vi "OpenLogs.vi"(8 "error in (no error)":errorcluster, 11 "object in":refnum<class "EventLogger_Actor.lvclass">) -> (0 "error out":errorcluster, 3 "object out":refnum<class "EventLogger_Actor.lvclass">)   [LabVIEW 2014, in "EventLogger_Actor.lvlib" / "EventLogger_Actor.lvclass"]
uses:
  EventLogger_Actor.lvclass
  EventLogger_Actor.lvclass/EventLogger_Actor.ctl
panel:
  # "Connector Pane"
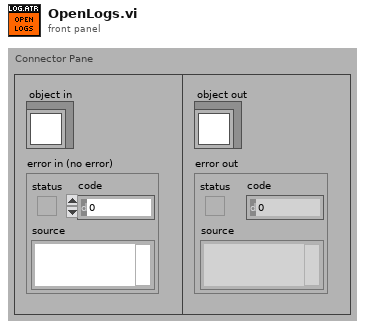
[diagram p1: front panel]
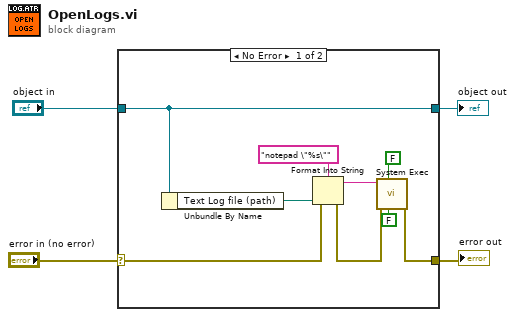
[diagram p0: block diagram]
diagram:
  n1 = case shown="No Error" "error in (no error)" {
    selector: "error in (no error)" -> [w13 w15]
    tunnel: [w11 w15] -> w3
    tunnel: [w12 w14] -> w1
    tunnel: "object in" -> [w12 w14]
    frame No Error {
      n2 = Unbundle By Name(w12) -> ("Text Log file (path)"=w5:path)
      n3 = Format Into String(format string="notepad \"%s\"", error in=w13, w5) -> (resulting string=w8:string, error out=w6:errorcluster)  [unwired: 1 in]
      n4 = call <vilib>:"System Exec.vi"("run minimized? (F)"=FALSE, "wait until completion? (T)"=FALSE, "error in (no error)"=w6, "command line"=w8) -> ("error out"=w11:errorcluster)  [unwired: 4 in, 3 out]
    }
    frame Error {
    }
  }
  "error out" <- w3
  "object out" <- w1
